vi "CfgFile Set Desc.vi"(8 "error in (no error)":errorcluster, 10 "UI Descriptions":T1, 11 "LF2R IDE in":refnum<class "LF2R IDE.lvclass">) -> (0 "error out":errorcluster, 3 "LF2R IDE out":refnum<class "LF2R IDE.lvclass">)   [LabVIEW 2018, in "LF2R IDE.lvlib" / "LF2R IDE.lvclass"]
uses:
  LF2R IDE.lvclass
  Const UI Description Setting.ctl
  Const UI Desc Frame Title.ctl
  Const UI Desc Property.ctl
  Const UI Desc Frame Basic.ctl
  Const UI Desc Frame Skill.ctl
  Const UI Desc Frame bp.ctl
  Const UI Desc Frame w.ctl
  Const UI Desc Frame b.ctl
  Const UI Desc Frame i.ctl
  Const UI Desc Frame o.ctl
  Const UI Desc Frame c.ctl
  Const UI Desc Other.ctl
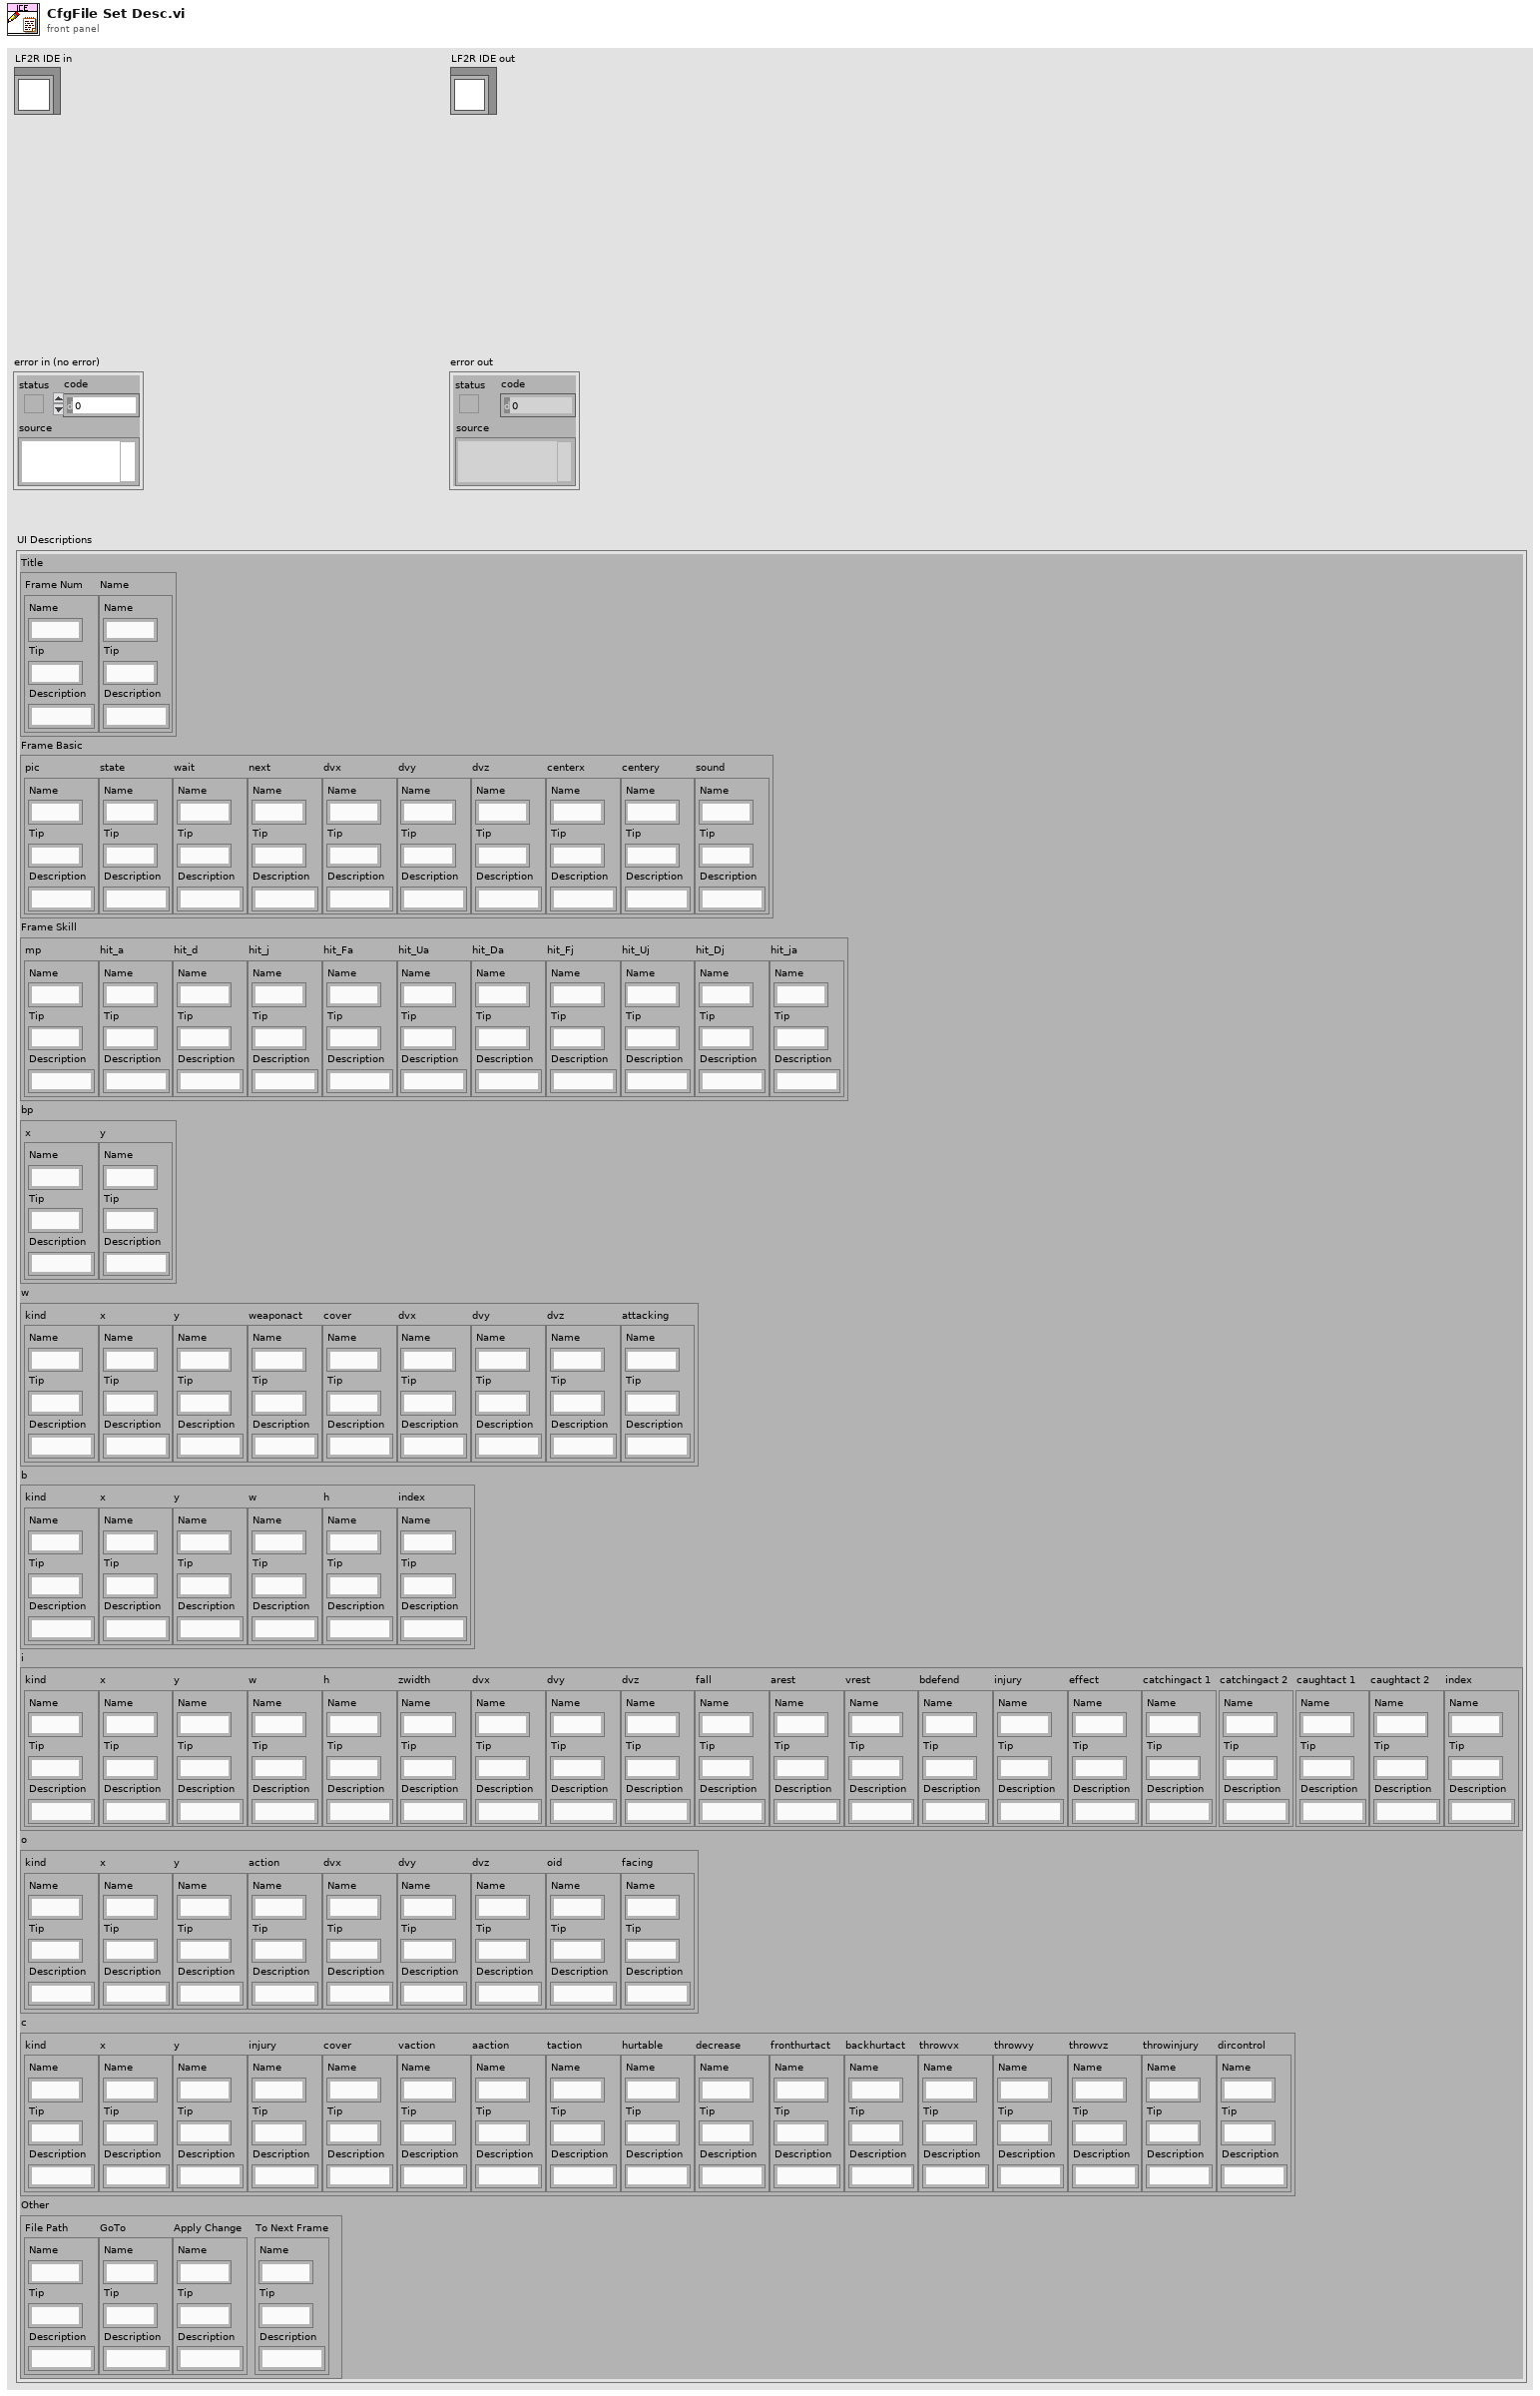
[diagram p1: front panel]
types:
  T1 = typedef "LF2R IDE.lvlib/LF2R IDE.lvclass/Const UI Description Setting.ctl" = cluster{"Title":T2, "Frame Basic":T4, "Frame Skill":T5, "bp":T6, "w":T7, "b":T8, "i":T9, "o":T10, "c":T11, "Other":T12}
  T2 = typedef "LF2R IDE.lvlib/LF2R IDE.lvclass/Const UI Desc Frame Title.ctl" = cluster{"Frame Num":T3, "Name":T3}
  T3 = typedef "LF2R IDE.lvlib/LF2R IDE.lvclass/Const UI Desc Property.ctl" = cluster{"Name":string, "Tip":string, "Description":string}
  T4 = typedef "LF2R IDE.lvlib/LF2R IDE.lvclass/Const UI Desc Frame Basic.ctl" = cluster{"pic":T3, "state":T3, "wait":T3, "next":T3, "dvx":T3, "dvy":T3, "dvz":T3, "centerx":T3, "centery":T3, "sound":T3}
  T5 = typedef "LF2R IDE.lvlib/LF2R IDE.lvclass/Const UI Desc Frame Skill.ctl" = cluster{"mp":T3, "hit_a":T3, "hit_d":T3, "hit_j":T3, "hit_Fa":T3, "hit_Ua":T3, "hit_Da":T3, "hit_Fj":T3, "hit_Uj":T3, "hit_Dj":T3, "hit_ja":T3}
  T6 = typedef "LF2R IDE.lvlib/LF2R IDE.lvclass/Const UI Desc Frame bp.ctl" = cluster{"x":T3, "y":T3}
  T7 = typedef "LF2R IDE.lvlib/LF2R IDE.lvclass/Const UI Desc Frame w.ctl" = cluster{"kind":T3, "x":T3, "y":T3, "weaponact":T3, "cover":T3, "dvx":T3, "dvy":T3, "dvz":T3, "attacking":T3}
  T8 = typedef "LF2R IDE.lvlib/LF2R IDE.lvclass/Const UI Desc Frame b.ctl" = cluster{"kind":T3, "x":T3, "y":T3, "w":T3, "h":T3, "index":T3}
  T9 = typedef "LF2R IDE.lvlib/LF2R IDE.lvclass/Const UI Desc Frame i.ctl" = cluster{"kind":T3, "x":T3, "y":T3, "w":T3, "h":T3, "zwidth":T3, "dvx":T3, "dvy":T3, "dvz":T3, "fall":T3, "arest":T3, "vrest":T3, "bdefend":T3, "injury":T3, "effect":T3, "catchingact 1":T3, "catchingact 2":T3, "caughtact 1":T3, "caughtact 2":T3, "index":T3}
  T10 = typedef "LF2R IDE.lvlib/LF2R IDE.lvclass/Const UI Desc Frame o.ctl" = cluster{"kind":T3, "x":T3, "y":T3, "action":T3, "dvx":T3, "dvy":T3, "dvz":T3, "oid":T3, "facing":T3}
  T11 = typedef "LF2R IDE.lvlib/LF2R IDE.lvclass/Const UI Desc Frame c.ctl" = cluster{"kind":T3, "x":T3, "y":T3, "injury":T3, "cover":T3, "vaction":T3, "aaction":T3, "taction":T3, "hurtable":T3, "decrease":T3, "fronthurtact":T3, "backhurtact":T3, "throwvx":T3, "throwvy":T3, "throwvz":T3, "throwinjury":T3, "dircontrol":T3}
  T12 = typedef "LF2R IDE.lvlib/LF2R IDE.lvclass/Const UI Desc Other.ctl" = cluster{"File Path":T3, "GoTo":T3, "Apply Change":T3, "To Next Frame":T3}
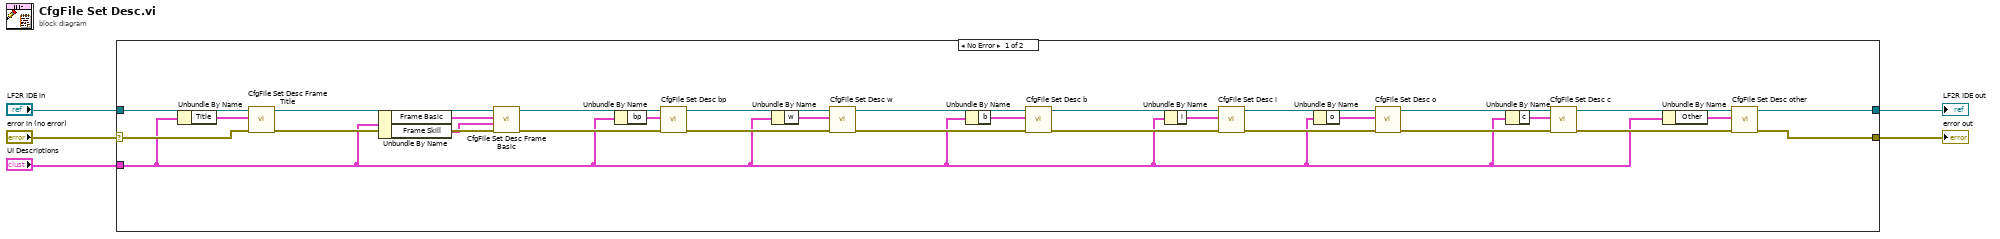
[diagram p0: block diagram]
diagram:
  n1 = case shown="No Error" "error in (no error)" {
    selector: "error in (no error)" -> [w34 w38]
    tunnel: [w6 w38] -> w4
    tunnel: [w7 w37] -> w2
    tunnel: "LF2R IDE in" -> [w36 w37]
    tunnel: "UI Descriptions" -> [w9 _]
    frame No Error {
      n2 = Unbundle By Name(w9) -> ("Title"=w35:T2)
      n3 = call "CfgFile Set Desc Frame Title.vi"("error in (no error)"=w34, "Title"=w35, "LF2R IDE in"=w36) -> ("error out"=w32:errorcluster, "LF2R IDE out"=w33:refnum<class "LF2R IDE.lvclass">)  [unwired: 7 in]
      n4 = Unbundle By Name(w9) -> ("Frame Basic"=w31:T4, "Frame Skill"=w30:T5)
      n5 = call "CfgFile Set Desc Frame Basic.vi"("error in (no error)"=w32, "Frame Skill"=w30, "Frame Basic"=w31, "LF2R IDE in"=w33) -> ("error out"=w28:errorcluster, "LF2R IDE out"=w29:refnum<class "LF2R IDE.lvclass">)  [unwired: 6 in]
      n6 = Unbundle By Name(w9) -> ("bp"=w27:T6)
      n7 = call "CfgFile Set Desc bp.vi"("error in (no error)"=w28, "bp"=w27, "LF2R IDE in"=w29) -> ("error out"=w25:errorcluster, "LF2R IDE out"=w26:refnum<class "LF2R IDE.lvclass">)  [unwired: 7 in]
      n8 = Unbundle By Name(w9) -> ("w"=w24:T7)
      n9 = call "CfgFile Set Desc w.vi"("error in (no error)"=w25, "w"=w24, "LF2R IDE in"=w26) -> ("error out"=w22:errorcluster, "LF2R IDE out"=w23:refnum<class "LF2R IDE.lvclass">)  [unwired: 7 in]
      n10 = Unbundle By Name(w9) -> ("b"=w21:T8)
      n11 = call "CfgFile Set Desc b.vi"("error in (no error)"=w22, "b"=w21, "LF2R IDE in"=w23) -> ("error out"=w19:errorcluster, "LF2R IDE out"=w20:refnum<class "LF2R IDE.lvclass">)  [unwired: 7 in]
      n12 = Unbundle By Name(w9) -> ("i"=w18:T9)
      n13 = call "CfgFile Set Desc i.vi"("error in (no error)"=w19, "i"=w18, "LF2R IDE in"=w20) -> ("error out"=w16:errorcluster, "LF2R IDE out"=w17:refnum<class "LF2R IDE.lvclass">)  [unwired: 7 in]
      n14 = Unbundle By Name(w9) -> ("o"=w13:T10)
      n15 = call "CfgFile Set Desc o.vi"("error in (no error)"=w16, "o"=w13, "LF2R IDE in"=w17) -> ("error out"=w14:errorcluster, "LF2R IDE out"=w15:refnum<class "LF2R IDE.lvclass">)  [unwired: 7 in]
      n16 = Unbundle By Name(w9) -> ("c"=w12:T11)
      n17 = call "CfgFile Set Desc c.vi"("error in (no error)"=w14, "c"=w12, "LF2R IDE in"=w15) -> ("error out"=w10:errorcluster, "LF2R IDE out"=w11:refnum<class "LF2R IDE.lvclass">)  [unwired: 7 in]
      n18 = Unbundle By Name(w9) -> ("Other"=w8:T12)
      n19 = call "CfgFile Set Desc other.vi"("error in (no error)"=w10, "Other"=w8, "LF2R IDE in"=w11) -> ("error out"=w6:errorcluster, "LF2R IDE out"=w7:refnum<class "LF2R IDE.lvclass">)  [unwired: 7 in]
    }
    frame Error {
    }
  }
  "error out" <- w4
  "LF2R IDE out" <- w2
